vi "thermo_check_status.vi"(11 "channel":T1={"type"=enum."COMET Tx5xx (ethernet)", "comment"="", "tag"="", "refresh"=5.0, "IP"="192.168.2.34", "port"=502, "VISA"="", "last readout"=timestamp(0 s since 1904-01-01), "TCP ref"=refnum, "VISA sess"="", "idn"="", "press"=0.0, "RH"=0.0, "temp"=0.0, "pres cor"=[], "RH cor"=[], "temp cor"=[], "try left"=0, "failed"=FALSE, "RTD set"=[], "RTD inv"=[], "range"=0.0, "net mode"=enum."MODBUS", "try fail"=enum."Stop trying - return NaN", "timeout [s]"=0.0, "max retries"=0} {"RTD inv" format="%.1f"; "RTD set" format="%.1f"; "temp cor" format="%.1f"; "RH cor" format="%.1f"; "pres cor" format="%.1f"; "refresh" min=0.1 max=1000.0 format="%.2f"}) -> (0 "fail or retry":bool, 1 "retry":bool, 2 "fail":bool, 3 "enabled":bool, 4 "retry N":i32=3 caption="try N" min=0 max=10, 6 "try":i32)   [LabVIEW 2020]
uses:
  thermo.ctl
  thermo_types.ctl
  Thermometer Fail Action.ctl
  thermo_var.vi
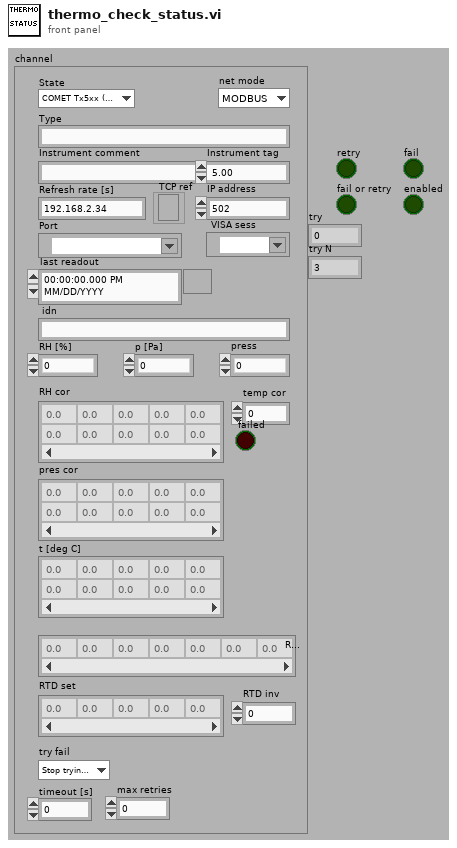
[diagram p1: front panel]
types:
  T1 = typedef "thermo.ctl" = cluster{"type":T2, "comment":string, "tag":string, "refresh":dbl, "IP":string, "port":u16, "VISA":refnum<visa-resource-name>, "last readout":timestamp, "TCP ref":refnum<k5>, "VISA sess":refnum<visa-resource-name>, "idn":string, "press":dbl, "RH":dbl, "temp":dbl, "pres cor":dbl[][], "RH cor":dbl[][], "temp cor":dbl[][], "try left":i32, "failed":bool, "RTD set":dbl[], "RTD inv":dbl[], "range":dbl, "net mode":enum16{"MODBUS", "HTTP"}, "try fail":T3, "timeout [s]":dbl, "max retries":i32}
  T2 = typedef "thermo_types.ctl" = enum16{"Disabled", "Simulated", "COMET Tx5xx (ethernet)", "Keithley 2002 (GPIB) + RTD", "Agilent 344xx (GPIB) + RTD"}
  T3 = typedef "Thermometer Fail Action.ctl" = enum16{"Stop trying - keep last value", "Stop trying - return NaN", "Generate error - stop sweep"}
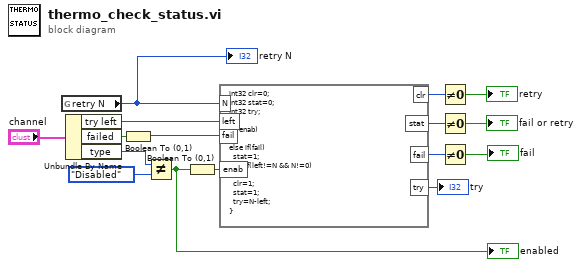
[diagram p0: block diagram]
diagram:
  n1 = global read "thermo_var.vi" "retry N"() -> (w15:i32)
  "retry N" <- w15
  n2 = Unbundle By Name("channel") -> ("try left"=w14:i32, "failed"=w16:bool, "type"=w4:T2)
  n3 = Boolean To (0,1)(Boolean=w16) -> (0, 1=w13:i16)
  n4 = Not Equal?(x=w4, y=thermo_types."Disabled") -> (x != y?=w2:bool)
  "enabled" <- w2
  n5 = Boolean To (0,1)(Boolean=w2) -> (0, 1=w1:i16)
  n6 = formula code="int32 clr=0;\nint32 stat=0;\nint32 try;\n\nif(!enab)\n  ;\nelse if(fail)\n  stat=1;\nelse if(left!=N && N!=0)\n{\n  clr=1;\n  stat=1;\n  try=N-left;\n}"("fail"=w13, "left"=w14, "N"=w15, "enab"=w1) -> ("stat"=w9:i32, "clr"=w12:i32, "fail"=w8:i16, "try"=→"try":i32)
  n7 = Not Equal To 0?(x=w12) -> (x != 0?=→"retry":bool)
  n8 = Not Equal To 0?(x=w9) -> (x != 0?=→"fail or retry":bool)
  n9 = Not Equal To 0?(x=w8) -> (x != 0?=→"fail":bool)
